vi "hamamatsuBufferIndexesOnly.vi"   [LabVIEW 2017]
uses:
  globalDevices.vi
  globalUtilities.vi
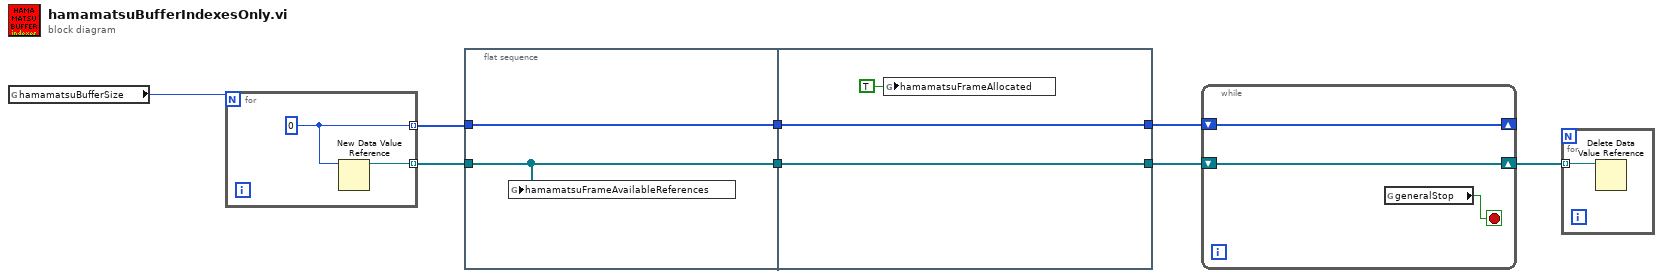
[diagram p0: block diagram]
diagram:
  n1 = global read "globalDevices.vi" "hamamatsuBufferSize"() -> (w8:i32)
  n2 = for {
    N: w8 -> [_]
    tunnel: [w10] -> w3 mode=indexing
    tunnel: [w9] -> w2 mode=indexing
    w10 = 0
    n3 = New Data Value Reference(data value=w10) -> (data value reference=w9:refnum<data-value>)  [unwired: 1 in, 1 out]
  }
  n4 = flat-sequence {
    tunnel: [w12] -> w7
    tunnel: w3 -> [w12]
    tunnel: w2 -> [w11]
    tunnel: [w11] -> w5
    tunnel: w7 -> [w14]
    tunnel: [w14] -> w6
    tunnel: w5 -> [w13]
    tunnel: [w13] -> w4
    frame #0 {
      n5 = global write "globalDevices.vi" "hamamatsuFrameAvailableReferences"(w11) -> ()
    }
    frame #1 {
      n6 = global write "globalDevices.vi" "hamamatsuFrameAllocated"(TRUE ("hamamatsuFrameAllocated")) -> ()
    }
  }
  n7 = while {
    shift-right: [w17] -> _
    shift-left: w6 -> [w17]
    shift-right: [w16] -> w1
    shift-left: w4 -> [w16]
    stop <- w18 stop-if-true
    n8 = global read "globalUtilities.vi" "generalStop"() -> (w18:bool)
  }
  n9 = for {
    tunnel: w1 -> [w19] mode=indexing
    n10 = Delete Data Value Reference(data value reference=w19) -> ()  [unwired: 1 in, 2 out]
  }
